vi "Audio-compression_tones.vi"() -> ()   [LabVIEW 2016]
doc: "This VI configures your sound card for both input and output. On a Macintosh, it could be the same device, while on Windows, it has to be different. Because of the delay of data buffering, it creates an effect of echoing."
uses:
  <vilib>/sound/lvsound.llb/Sound Format.ctl
  <vilib>/sound2/lvsound2.llb/Sound Data Format.ctl
  <vilib>/Platform/TimedLoop/XDataNode/timing_clust.ctl
  <vilib>/Platform/TimedLoop/XDataNode/nitl_modes.ctl
  <vilib>/Platform/TimedLoop/XDataNode/wakeup.ctl
  <vilib>/Analysis/4window.llb/Cosine Tapered Window (DBL).vi
  <vilib>/Analysis/3filter.llb/Butterworth Filter (DBL).vi
  <vilib>/measure/matone.llb/Extract Multiple Tone Information 1 Chan.vi
  <vilib>/sound2/lvsound2.llb/Sound Output Write (DBL Single).vi
  <vilib>/Platform/TimedLoop/XDataNode/XDataNode.xnode
  <vilib>/Platform/TimedLoop/XDataNode/XDNodeRunTimeDep.lvlib
  <vilib>/measure/NI_MAPro.lvlib
  <vilib>/Analysis/NI_AALBase.lvlib
  <vilib>/Analysis/NI_AALPro.lvlib
panel:
  in  "Audio File":string="marching_illini.wav"
  out "Sound format rate\n(samples/sec)":i32
  in  "device ID":u32
  in  "Hear original\nor Compressed?":bool
  out "msec":i64
  in  "Block size (Samples)":i32=4096
  out "Finished Late? [i-1]":bool
  out "Compression Factor (Ratio):":dbl
  out "Original # of Sound Samples:":i32
  in  "Number of Tones (Sinusoids) to Use":i32(ring)=25 items=["1 Sinusoids"=1, "2 Sinusoids"=2, "3 Sinusoids"=3, "4 Sinusoids"=4, "5 Sinusoids"=5, "6 Sinusoids"=6, "7 Sinusoids"=7, "8 Sinusoids"=8, "9 Sinusoids"=9, "10 Sinusoids"=10, "15 Sinusoids"=15, "20 Sinusoids"=20, "25 Sinusoids"=25]
  out "Phase":dbl[](array[numeric])
  out "Amplitude":dbl[](array[numeric])
  out "Frequency":dbl[](array[numeric])
  in  "Stop":bool
  out "sound format":T1
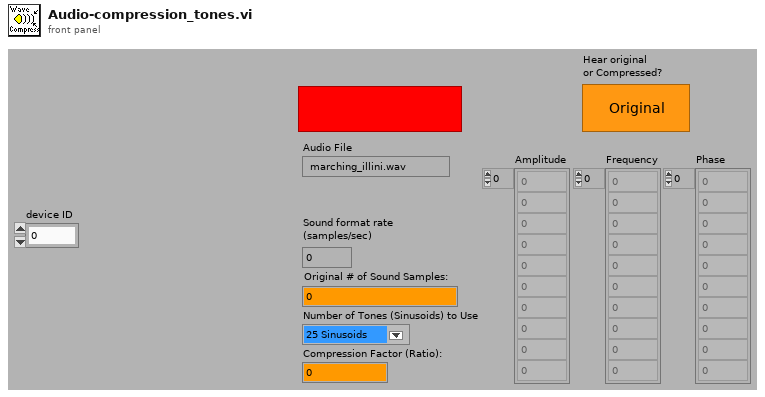
[diagram p1: front panel]
types:
  T1 = typedef "Sound Format.ctl" = cluster{"sound quality":enum16{"mono", "stereo"}, "rate":enum16{"11025", "22050", "44100", "8000"}, "bits per sample":enum16{"8 bit", "16 bit"}}
  T2 = typedef "Sound Data Format.ctl" = cluster{"sample rate (S/s)":dbl, "number of channels":i32, "bits per sample":i32}
  T3 = typedef "Sound Output Task ID.ctl" = u32
  T4 = typedef "XDNodeRunTimeDep.lvlib/timing_clust.ctl" = cluster{"Expected End [f-1]":u64, "Actual End [f-1]":u64, "Finished Late? [f-1]":bool, "Expected End [i-1]":u64, "Actual End [i-1]":u64, "Finished Late? [i-1]":bool, "Expected Start [i]":u64, "Actual Start [i]":u64, "Expected Start [f]":u64, "Actual Start [f]":u64, "Source Name":string, "Structure Name":string, "Period":i64, "Deadline":i64, "Offset":i64, "Start":i64, "Priority":i32, "Timeout":i32, "Mode":T5, "Wakeup Reason":T6, "Error":errorcluster, "Source Type":string, "Secondary Source Type":string, "Global End Time":u64, "Global Start Time":u64, "Frame Duration":u64, "Iteration Duration":u64, "Assigned CPU":i32, "I/O Scan Engine Mode":u32}
  T5 = typedef "XDNodeRunTimeDep.lvlib/nitl_modes.ctl" = enum32{"No Change", "Process missed periods, maintain original phase", "Discard missed periods, maintain original phase", "Process missed periods, ignore original phase", "Discard missed periods, ignore original phase"}
  T6 = typedef "XDNodeRunTimeDep.lvlib/wakeup.ctl" = enum32{"Normal", "Aborted", "Asynchronous wakeup", "Timing source error", "Timed loop error", "Timeout"}
  T7 = enum32{"Lowpass", "Highpass", "Bandpass", "Bandstop"}
  T8 = cluster{"detected frequency":dbl, "detected amplitude":dbl, "detected phase (deg)":dbl}[]
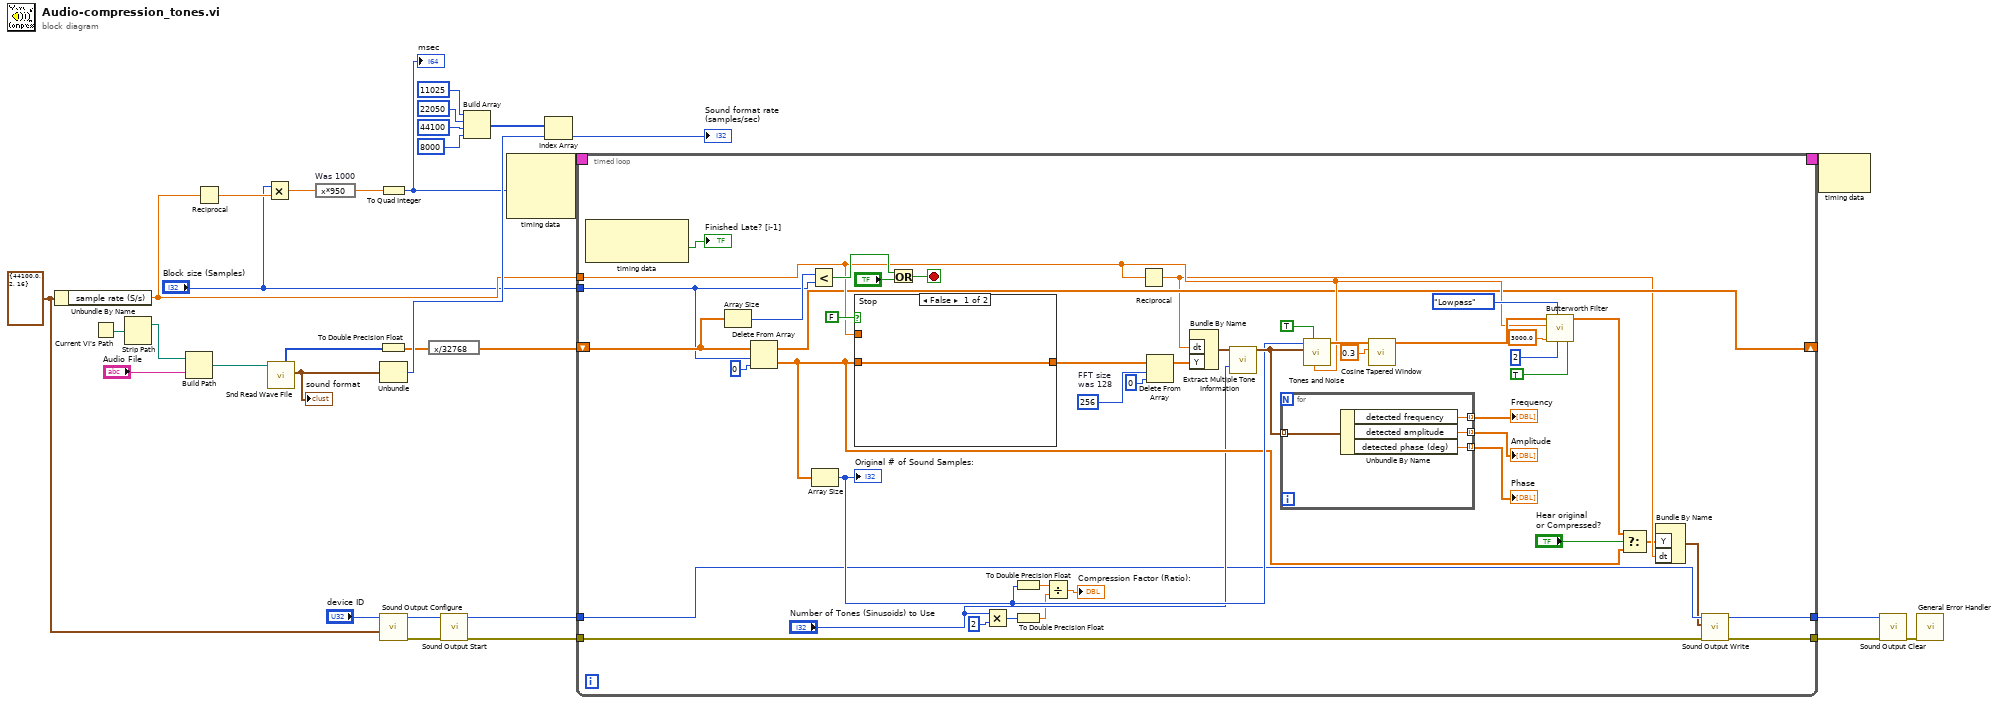
[diagram p0: block diagram]
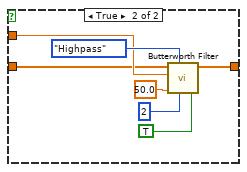
[diagram p2: hidden frame]
diagram:
  w15 = T2 {"sample rate (S/s)"=44100.0, "number of channels"=2, "bits per sample"=16} ("sound format")
  n1 = Unbundle By Name(w15) -> ("sample rate (S/s)"=w12:dbl)
  n2 = Current VI's Path() -> (path=w4:path)
  n3 = Strip Path(path=w4) -> (stripped path=w1:path)  [unwired: 1 out]
  n4 = Build Path(base path=w1, name or relative path="Audio File") -> (appended path=w2:path)
  n5 = Reciprocal(x=w12) -> (1/x=w20:dbl)
  n6 = Multiply(x="Block size (Samples)", y=w20) -> (x*y=w19:dbl)
  n7 = call <vilib>:"Snd Read Wave File.vi"("wave file path"=w2) -> ("sound format"=w32:T1, "mono 16-bit"=w9:i16[])  [unwired: 1 in, 8 out]
  "sound format" <- w32
  n8 = expression code="x*950" "Was 1000"(w19) -> (w10:dbl)
  n9 = To Quad Integer(1:w10) -> (0:w5:i64)
  "msec" <- w5
  n10 = To Double Precision Float(number=w9) -> (double precision float=w7:dbl[])
  n11 = Unbundle(w32) -> ("rate"=w25:enum16{"11025", "22050", "44100", "8000"})  [unwired: 2 out]
  n12 = call <vilib>:"Sound Output Configure.vi"("sound format"=w15, "device ID"="device ID") -> ("error out"=w16:errorcluster, "task ID"=w17:T3)  [unwired: 8 in]
  n13 = expression code="x/32768"(w7) -> (w8:dbl[])
  n14 = call <vilib>:"Sound Output Start.vi"("error in (no error)"=w16, "task ID"=w17) -> ("error out"=w13:errorcluster, "task ID out"=w14:T3)  [unwired: 8 in]
  n15 = Build Array(11025 ("element"), 22050 ("element"), 44100 ("element"), 8000 ("element")) -> (w26:i32[])
  n16 = node-c288(w5) -> (w21:T4)  [unwired: 2 out]
  n17 = Index Array(array=w26, index=w25) -> (element=→"Sound format rate\n(samples/sec)":i32)
  n18 = timed-loop {
    tunnel: w12 -> [w53]
    tunnel: "Block size (Samples)" -> [w51]
    tunnel: [w43] -> w29
    tunnel: [w42] -> w30
    tunnel: w13 -> [w45]
    tunnel: w14 -> [w44]
    shift-left: w8 -> [w76]
    shift-right: [w47] -> _
    timing-out: [_] -> w22
    timing: w21 -> [_]
    stop <- w72 stop-if-true
    w70 = 256  # FFT size was 128
    n19 = node-c288() -> (→"Finished Late? [i-1]":bool)  [unwired: 2 out]
    n20 = Array Size(array=w76) -> (size(s)=w75:i32)
    n21 = Delete From Array(array=w76, length=w51, index=0) -> (deleted portion=w48:dbl[], array with subset deleted=w47:dbl[])
    n22 = Less?(x=w75, y=w51) -> (x < y?=w73:bool)
    n23 = Array Size(array=w48) -> (size(s)=w54:i32)
    "Original # of Sound Samples:" <- w54
    n24 = case shown="False" FALSE {
      tunnel: [w82 w85] -> w50
      tunnel: w53 -> [_ w84]
      tunnel: w48 -> [w82 w83]
      frame False {
      }
      frame True {
        n25 = call-poly <vilib>:"Butterworth Filter.vi"("init/cont (init:F)"=TRUE, "order"=2, "filter type"=T7."Highpass", "low cutoff freq: fl"=50.0, "sampling freq: fs"=w84, "X"=w83) -> ("Filtered X"=w85:dbl[])  [unwired: 1 in, 2 out]
      }
    }
    n26 = Or(x=w73, y="Stop") -> (x .or. y?=w72:bool)
    n27 = Multiply(x="Number of Tones (Sinusoids) to Use", y=2) -> (x*y=w66:i32)
    n28 = To Double Precision Float(number=w54) -> (double precision float=w37:dbl)
    n29 = To Double Precision Float(number=w66) -> (double precision float=w36:dbl)
    n30 = Divide(x=w37, y=w36) -> (x/y=→"Compression Factor (Ratio):":dbl)
    n31 = Reciprocal(x=w53) -> (1/x=w40:dbl)
    n32 = Delete From Array(array=w50, length=w70, index=0) -> (array with subset deleted=w69:dbl[])  [unwired: 1 out]
    n33 = Bundle By Name("dt"=w40, "Y"=w69) -> (w64:waveform(dbl))  [unwired: 1 out]
    n34 = call-poly <vilib>:"Extract Multiple Tone Information.vi"("time signal in"=w64, "max num tones"="Number of Tones (Sinusoids) to Use") -> ("multiple tone information"=w57:T8)  [unwired: 4 in, 9 out]
    n35 = for {
      tunnel: w57 -> [w79] mode=indexing
      tunnel: [w78] -> w33 mode=indexing
      tunnel: [w81] -> w34 mode=indexing
      tunnel: [w80] -> w35 mode=indexing
      n36 = Unbundle By Name(w79) -> ("detected frequency"=w78:dbl, "detected amplitude"=w81:dbl, "detected phase (deg)"=w80:dbl)
    }
    "Frequency" <- w33
    "Amplitude" <- w34
    "Phase" <- w35
    n37 = call <vilib>:"Tones and Noise.vi"("Fs"=w53, "reset signal"=TRUE, "tones"=w57, "samples"=w54) -> ("tones and noise"=w63:dbl[])  [unwired: 3 in, 4 out]
    n38 = call-poly <vilib>:"Cosine Tapered Window.vi"("ratio"=0.3, "X"=w63) -> ("Windowed X"=w62:dbl[])  [unwired: 9 out]
    n39 = call-poly <vilib>:"Butterworth Filter.vi"("init/cont (init:F)"=TRUE, "order"=2, "filter type"=T7."Lowpass", "low cutoff freq: fl"=3000.0, "sampling freq: fs"=w53, "X"=w62) -> ("Filtered X"=w38:dbl[])  [unwired: 1 in, 2 out]
    n40 = Select(t=w38, s="Hear original\nor Compressed?", f=w48) -> (s? t:f=w39:dbl[])
    n41 = Bundle By Name("Y"=w39, "dt"=w40) -> (w41:waveform(dbl))  [unwired: 1 in]
    n42 = call-poly <vilib>:"Sound Output Write.vi"("error in (no error)"=w45, "data"=w41, "task ID"=w44) -> ("error out"=w42:errorcluster, "task ID out"=w43:T3)  [unwired: 7 in]
  }
  n43 = node-c288(w22) -> ()  [unwired: 1 out]
  n44 = call <vilib>:"Sound Output Clear.vi"("error in (no error)"=w30, "task ID"=w29) -> ("error out"=w31:errorcluster)  [unwired: 9 in]
  n45 = call <vilib>:"General Error Handler.vi"("error in (no error)"=w31) -> ()  [unwired: 2 in, 13 out]
